vi "Set Auxiliary Amplifier Mode.vi"(8 "error in (no error)":errorcluster, 10 "Amplifier Mode (F: Off)":bool, 11 "VISA resource name":refnum<visa-resource-name>) -> (0 "error out":errorcluster, 3 "VISA resource name out":refnum<visa-resource-name>)   [LabVIEW 2014, in "Fluke 5XXX Series Multicalibrators.lvlib"]
doc: "This VI activate or deactivate an auxiliary amplifier and set the source preference to this amplifier or to the calibrator.\n\nNotes:\n\n(1) An error is reported if the auxiliary amplifier cannot be turned on or off for the present output.\n\n(2) Instrument model 5520A and 57LFC can not use auxiliary amplifier."
uses:
  Fluke 5XXX Series Multicalibrators.lvlib
panel:
  # "On"
  # "Off"
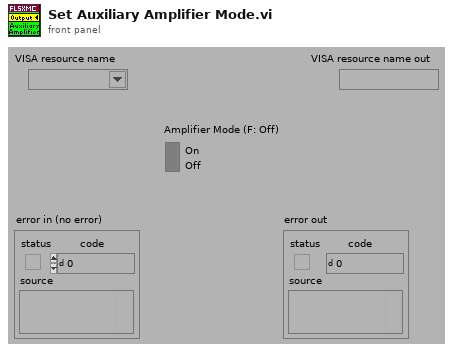
[diagram p1: front panel]
types:
  T1 = cluster{"Status":bool, "Code":i32, "Source (VI Name)":string}
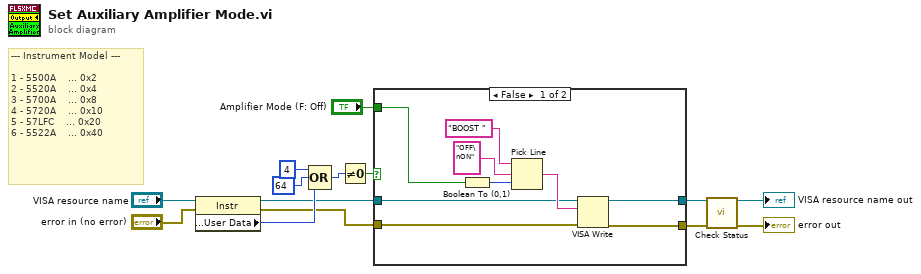
[diagram p0: block diagram]
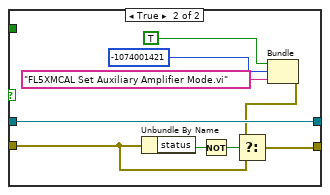
[diagram p2: hidden frame]
diagram:
  # "--- Instrument Model ---\n\n1 - 5500A    ... 0x2\n2 - 5520A    ... 0x4\n3 - 5700A    ... 0x8\n4 - 5720A    ... 0x10\n5 - 57LFC    ... 0x20\n6 - 5522A    ... 0x40"
  n1 = property class="Instr"(reference="VISA resource name", error in="error in (no error)") -> (reference out=w4:refnum<visa-resource-name>, error out=w3:errorcluster, "General Settings:User Data"=w8:u32)
  n2 = Compound Arithmetic op=OR(u32 4 ("Numeric"), 64 ("Numeric"), w8) -> (w7:u32)
  n3 = Not Equal To 0?(x=w7) -> (x != 0?=w2:bool)
  n4 = case shown="False" w2 {
    tunnel: "Amplifier Mode (F: Off)" -> [w20 _]
    tunnel: [w18 w29] -> w11
    tunnel: [w19 w24] -> w10
    tunnel: w4 -> [w16 w29]
    tunnel: w3 -> [w15 w26]
    frame False {
      n5 = Boolean To (0,1)(Boolean=w20) -> (0, 1=w21:i16)
      n6 = Pick Line(string ("")="BOOST " ("Reset Command"), multi-line string="OFF\nON", line index=w21) -> (output string=w17:string)
      n7 = VISA Write(VISA resource name=w16, write buffer=w17, error in (no error)=w15) -> (VISA resource name out=w18:refnum<visa-resource-name>, error out=w19:errorcluster)  [unwired: 1 out]
    }
    frame True {
      n8 = Unbundle By Name(w26) -> ("status"=w28:bool)
      n9 = Not(x=w28) -> (.not. x?=w27:bool)
      n10 = Bundle("Status"=TRUE, "Code"=-1074001421, "Source (VI Name)"="FL5XMCAL Set Auxiliary Amplifier Mode.vi") -> (w25:T1)  [unwired: 1 in]
      n11 = Select(t=w25, s=w27, f=w26) -> (s? t:f=w24:errorcluster)
    }
  }
  n12 = call "Check Status.vi"("VISA resource name"=w11, "error in (no error)"=w10) -> ("VISA resource name out"=→"VISA resource name out":refnum<visa-resource-name>, "error out"=→"error out":errorcluster)  [unwired: 12 in]
